vi "VFRDA Volumetric Flow Rate of Dry Air (m3 to S).vi"(1 "Gas Presure":dbl[unit]=80000.0 min=80000.0 max=120000.0, 2 "Tceg":dbl[unit], 3 "MFRHA\nMass Flow Rate of Humid Air (Kg/s)":dbl[unit], 4 "RH":dbl) -> (0 "VFRDA":dbl[unit])   [LabVIEW 2018]
panel:
  out "VFRDA\nVolumetric Flow Rate of Dry Air\nVFRDA=MFRDA/PDDA;":dbl[unit](knob) scale=0.0..10.0
  out "Temprature Of Input Air\nKelvin Degree":dbl[unit](slide) scale=273.0..373.0
  out "Tk":dbl[unit]
  out "Temprature Of Input Air\nCentigrade Degree":dbl[unit](slide) scale=0.0..100.0
  out "Humidity of Input Air":dbl(knob) scale=0.0..100.0
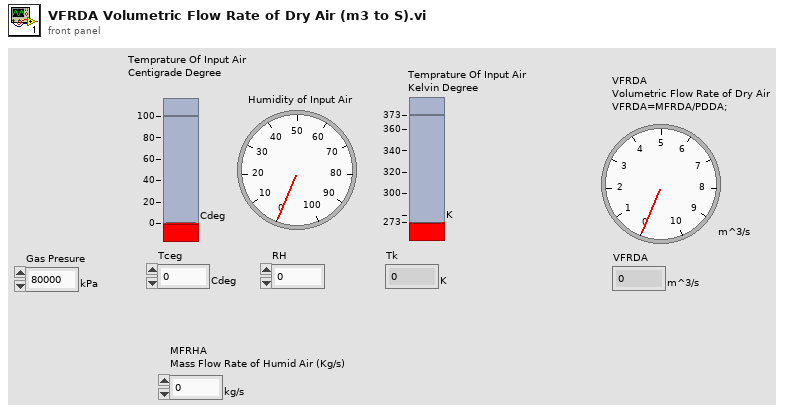
[diagram p1: front panel]
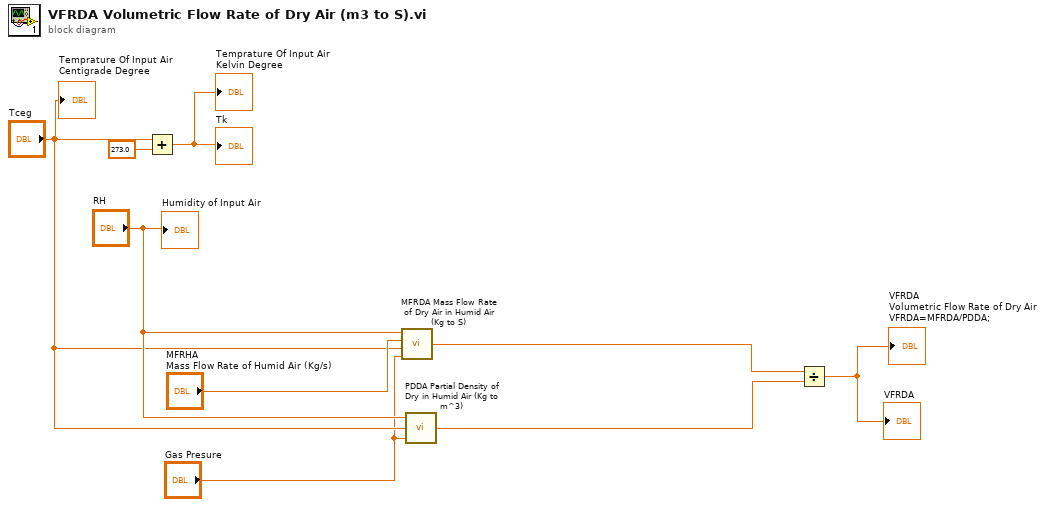
[diagram p0: block diagram]
diagram:
  n1 = Add(x="Tceg", y=dbl[unit] 273.0) -> (x+y=→"Tk" →"Temprature Of Input Air\nKelvin Degree":dbl[unit])
  n2 = call "MFRDA Mass Flow Rate of Dry Air in Humid Air (Kg to S).vi"("Gas Presure"="Gas Presure", "Tceg"="Tceg", "MFRHA\nMass Flow Rate of Humid Air (Kg/s)"="MFRHA\nMass Flow Rate of Humid Air (Kg/s)", "RH"="RH") -> ("MFRDA"=w4:dbl[unit])
  n3 = call "PDDA Partial Density of Dry in Humid Air (Kg to m^3).vi"("Total Pressure of Humid Air"="Gas Presure", "Tceg"="Tceg", "RH"="RH") -> ("PDDA"=w6:dbl[unit])
  n4 = Divide(x=w4, y=w6) -> (x/y=→"VFRDA\nVolumetric Flow Rate of Dry Air\nVFRDA=MFRDA/PDDA;" →"VFRDA":dbl[unit])
  "Humidity of Input Air" <- "RH"
  "Temprature Of Input Air\nCentigrade Degree" <- "Tceg"
